vi "Write New Pose.vi"(8 "error in (no error)":errorcluster, 10 "New Pose?":bool, 11 "UR5 Robot in":refnum<class "UR5 Robot.lvclass">) -> (0 "error out":errorcluster, 3 "UR5 Robot out":refnum<class "UR5 Robot.lvclass">)   [LabVIEW 2018, in "UR5 Robot.lvlib" / "UR5 Robot.lvclass"]
uses:
  UR5 Robot.lvclass
  UR5 Robot.lvclass/UR5 Robot.ctl
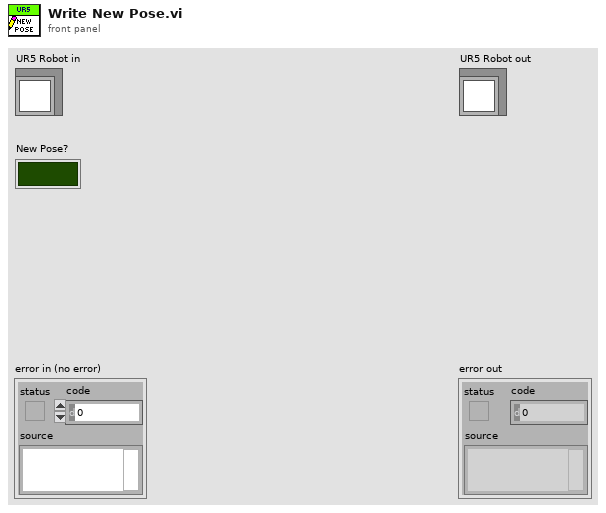
[diagram p1: front panel]
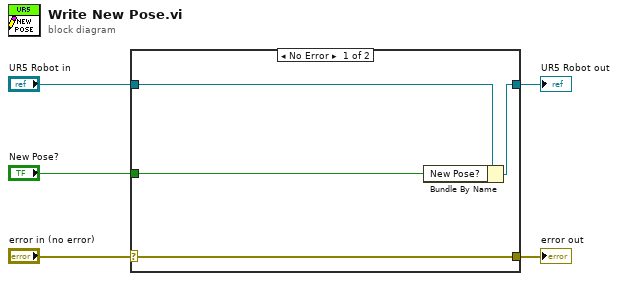
[diagram p0: block diagram]
diagram:
  n1 = case shown="No Error" "error in (no error)" {
    selector: "error in (no error)" -> [w9 w10]
    tunnel: [w9 w10] -> w4
    tunnel: [w7 w11] -> w2
    tunnel: "UR5 Robot in" -> [w8 w11]
    tunnel: "New Pose?" -> [w6 _]
    frame No Error {
      n2 = Bundle By Name(cluster=w8, "New Pose?"=w6) -> (w7:refnum<class "UR5 Robot.lvclass">)
    }
    frame Error {
    }
  }
  "error out" <- w4
  "UR5 Robot out" <- w2
